vi "test.vi"() -> ()   [LabVIEW 2020]
panel:
  out "数组":dbl[](array[numeric])
  in  "测量队列":T1(array[cluster])
  in  "确定按钮":bool
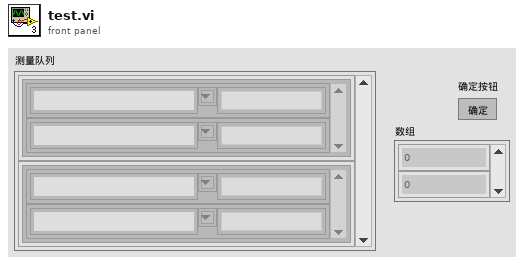
[diagram p1: front panel]
types:
  T1 = cluster{"测量参数":cluster{"设置项":string, "值":string}[]}[]
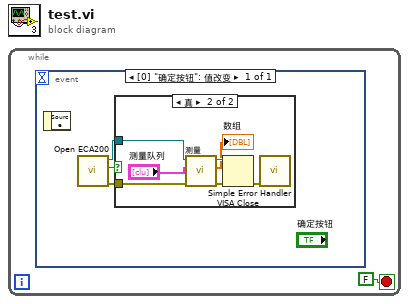
[diagram p0: block diagram]
diagram:
  n1 = while {
    stop <- FALSE stop-if-true
    n2 = event shown="[0] \"确定按钮\": 值改变" {
      selector: _ -> [_]
      dyn-events: _ -> [_]
      timeout: _ -> [_]
      event "确定按钮": Value Change {
        n3 = event-data() -> ()  [unwired: 1 in, 1 out]
        n4 = call "Open ECA200.vi"() -> ("错误输出"=w3:errorcluster, "仪器存在"=w4:bool, "VISA资源名称输出"=w2:refnum<visa-resource-name>)  [unwired: 9 in]
        n5 = case shown="真" w4 {
          tunnel: w3 -> [_ w11]
          tunnel: w2 -> [_ w10]
          frame False {
          }
          frame True {
            n6 = call "测量.vi"("错误输入（无错误）"=w11, "测量队列"="测量队列", "VISA资源名称"=w10) -> ("错误输出"=w9:errorcluster, "数组"=→"数组":dbl[], "VISA资源名称输出"=w8:refnum<visa-resource-name>)  [unwired: 6 in]
            n7 = VISA Close(VISA resource name=w8, error in (no error)=w9) -> (error out=w7:errorcluster)
            n8 = call <vilib>:"Simple Error Handler.vi"("error in (no error)"=w7) -> ()  [unwired: 4 in, 5 out]
          }
        }
      }
    }
  }
